vi "Zero Velocity.vi"   [LabVIEW 2015]
uses:
  _TypeDefs/Z900_navX_ActionTypeDef.ctl
types:
  T1 = typedef "Z900_navX_ActionTypeDef.ctl" = enum16{"None", "Halt", "Normal Read", "Update Serial Protocol", "Update Rate Htz", "Zero-Yaw", "Zero-Displacement", "Zero-Velocity"}
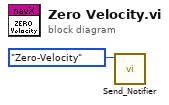
[diagram p0: block diagram]
diagram:
  n1 = call "Send_Notifier.vi"("navX Action"=Z900_navX_ActionTypeDef."Zero-Velocity") -> ()  [unwired: 11 in]
